vi "Update Position.vi"(8 "error in (no error)":errorcluster, 9 "Position (0:4)":i32, 10 "Filter Wheel (0:n-1)":i32, 11 "Filter Wheel in":refnum<class "Filter Wheel.lvclass">) -> (0 "error out":errorcluster, 3 "Filter Wheel out":refnum<class "Filter Wheel.lvclass">)   [LabVIEW 2024, in "Filter Wheel.lvclass"]
uses:
  Filter Wheel.lvclass
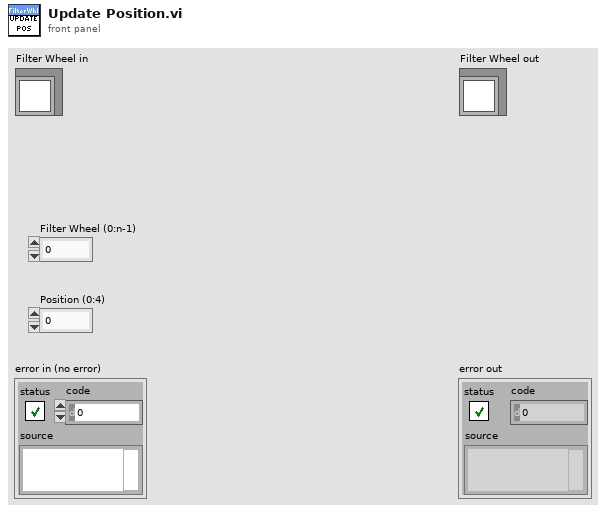
[diagram p1: front panel]
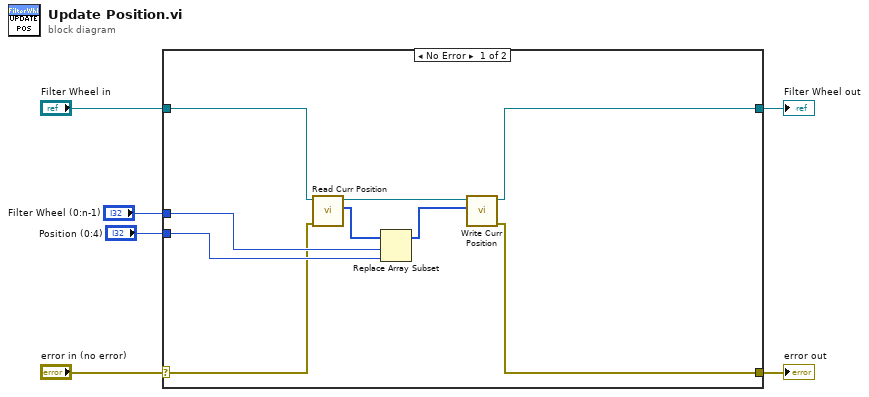
[diagram p0: block diagram]
diagram:
  n1 = case shown="No Error" "error in (no error)" {
    selector: "error in (no error)" -> [w8 w17]
    tunnel: [w7 w17] -> w5
    tunnel: [w10 w16] -> w3
    tunnel: "Filter Wheel in" -> [w9 w16]
    tunnel: "Filter Wheel (0:n-1)" -> [w14 _]
    tunnel: "Position (0:4)" -> [w13 _]
    frame No Error {
      n2 = call-dynamic "Read Curr Position.vi"("error in (no error)"=w8, "Filter Wheel in"=w9) -> ("Curr Position"=w15:i32[], "Filter Wheel out"=w11:refnum<class "Filter Wheel.lvclass">)  [unwired: 7 in, 1 out]
      n3 = Replace Array Subset(array=w15, new element=w13, index=w14) -> (w12:i32[])
      n4 = call-dynamic "Write Curr Position.vi"("Curr Position"=w12, "Filter Wheel in"=w11) -> ("error out"=w7:errorcluster, "Filter Wheel out"=w10:refnum<class "Filter Wheel.lvclass">)  [unwired: 8 in]
    }
    frame Error {
    }
  }
  "error out" <- w5
  "Filter Wheel out" <- w3
